vi "界面UI.vi"() -> ()   [LabVIEW 2016, in "科盛超标留样.lvlib"]
uses:
  <vilib>/Utility/miscctls.llb/LVPointTypeDef.ctl
panel:
  in  "当前解析模式":string(combo)
  in  "切换串口":bool
  out "查询系统状态":T1
  out "查询瓶记录":T2
  out "输出数组":T3(array[cluster])
  in  "留样命令":bool
  in  "供样命令":bool
  in  "触发采样":bool
  in  "查询系统状态":bool
  in  "远程取样":bool
  in  "复位指令":bool
  in  "查询瓶记录":bool
  in  "查询采样记录":bool
  in  "VISA resource name":refnum<visa-resource-name>="COM2" caption="VISA资源名称"
  in  "写入缓冲区":string
  out "读取缓冲区":string
  out "source":string
  out "通讯":bool
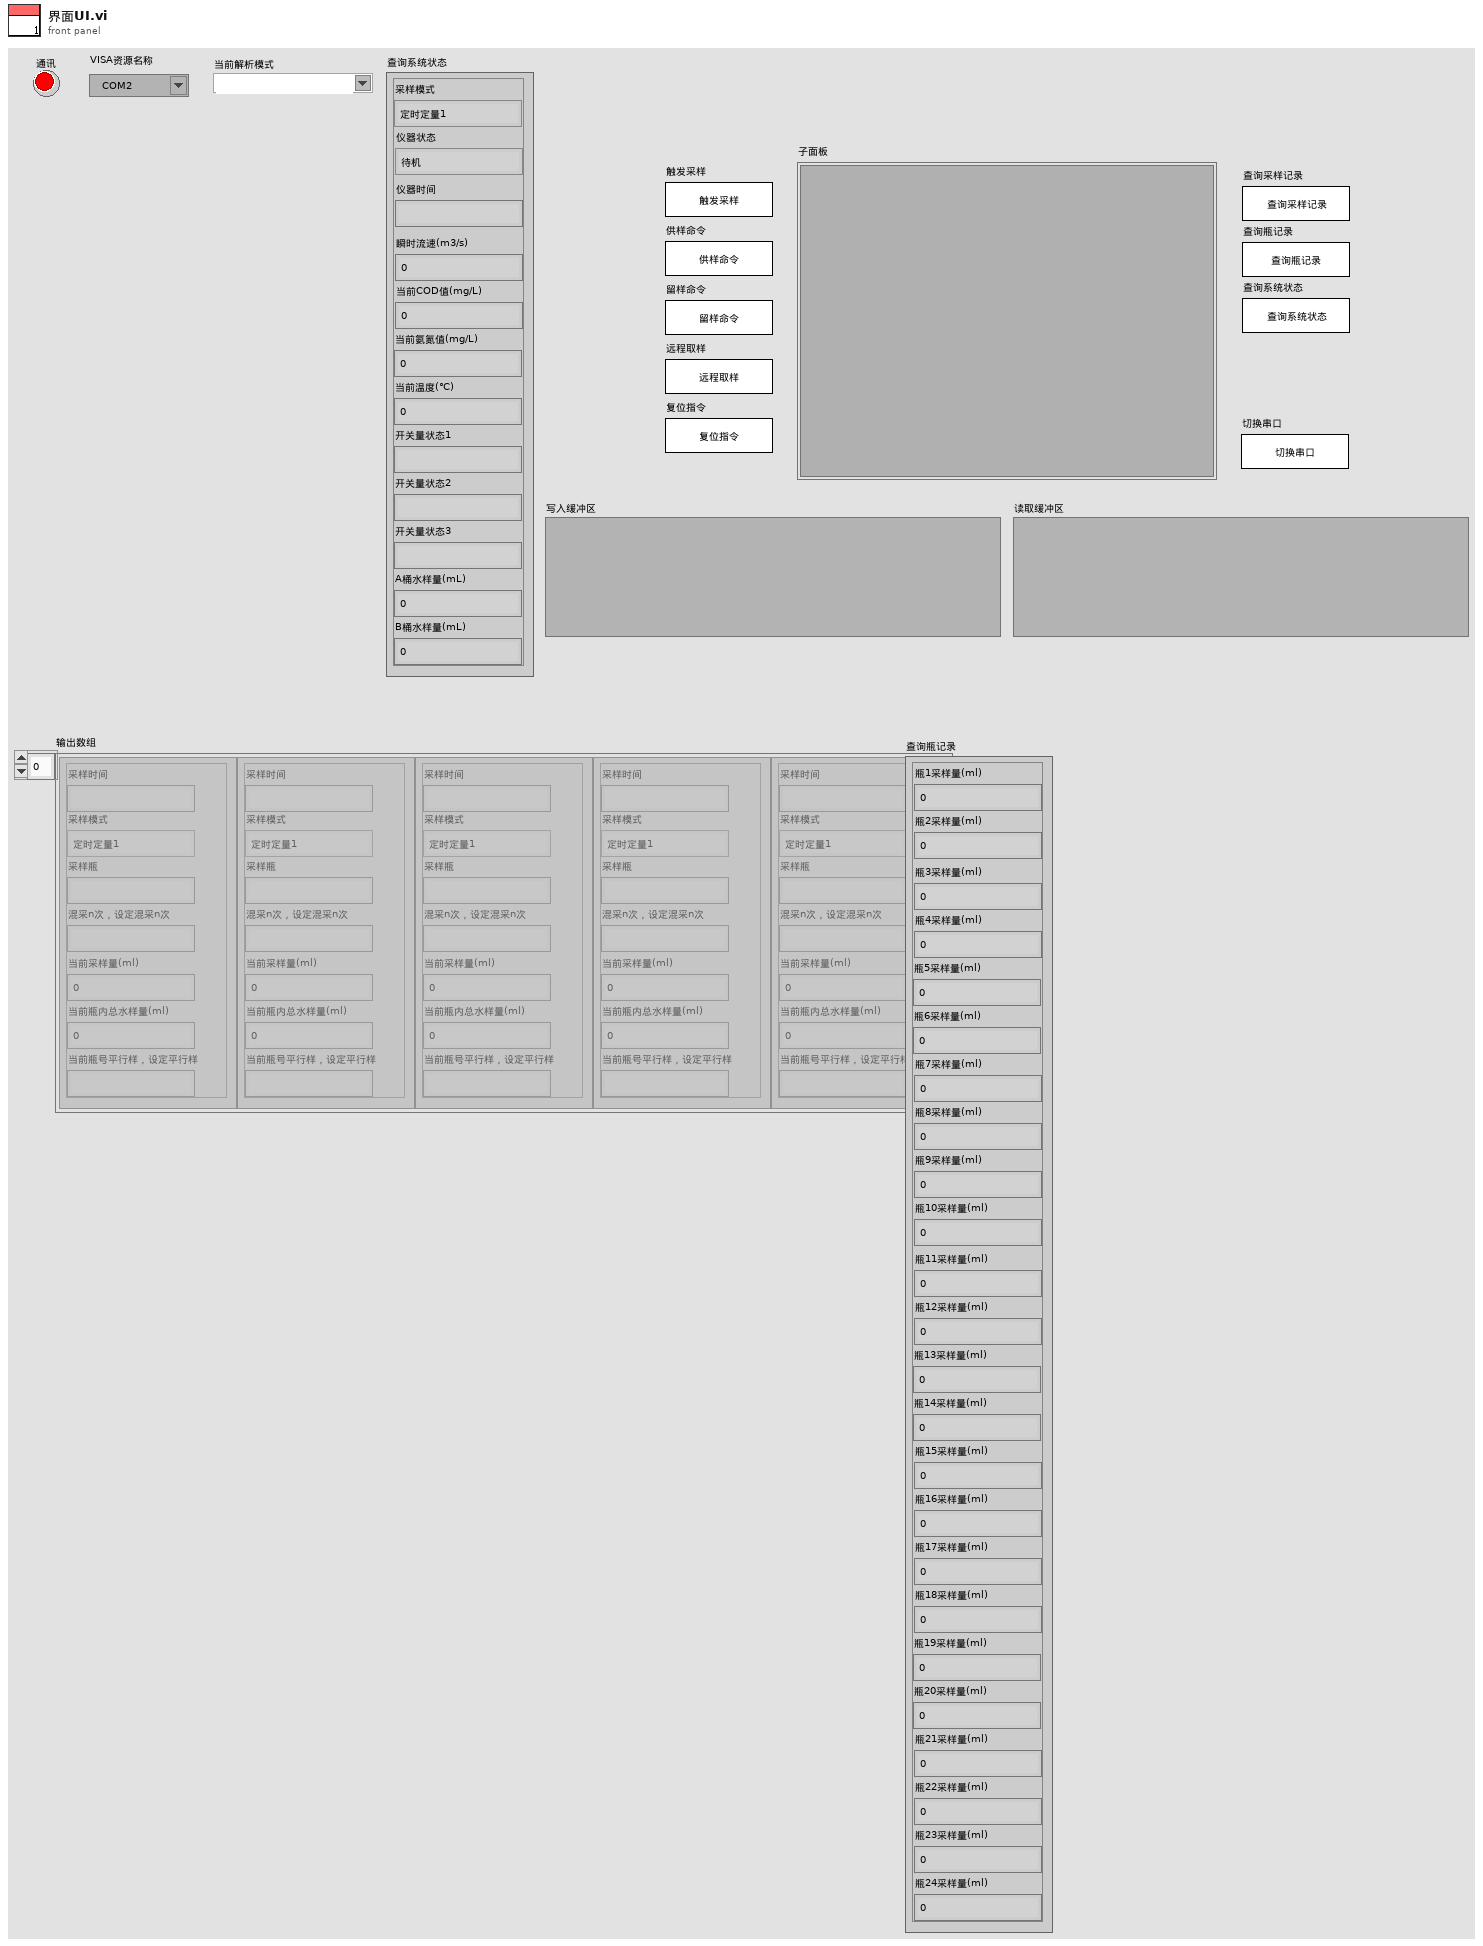
[diagram p1: front panel]
types:
  T1 = cluster{"采样模式":enum16{"定时定量1", "定时定量2", "定流定量", "定时比例", "同步留样", "超标留样", "触发采样", "定时采样1", "定流供样", "定时采样2", "远程取样", "手动取样", "流量跟踪"}, "仪器状态":enum16{"待机", "运行中"}, "仪器时间":string, "瞬时流速(m3/s)":dbl, "当前COD值(mg/L)":dbl, "当前氨氮值(mg/L)":dbl, "当前温度(℃)":dbl, "开关量状态1":string, "开关量状态2":string, "开关量状态3":string, "A桶水样量(mL)":dbl, "B桶水样量(mL)":dbl}
  T2 = cluster{"瓶1采样量(ml)":dbl, "瓶2采样量(ml)":dbl, "瓶3采样量(ml)":dbl, "瓶4采样量(ml)":dbl, "瓶5采样量(ml)":dbl, "瓶6采样量(ml)":dbl, "瓶7采样量(ml)":dbl, "瓶8采样量(ml)":dbl, "瓶9采样量(ml)":dbl, "瓶10采样量(ml)":dbl, "瓶11采样量(ml)":dbl, "瓶12采样量(ml)":dbl, "瓶13采样量(ml)":dbl, "瓶14采样量(ml)":dbl, "瓶15采样量(ml)":dbl, "瓶16采样量(ml)":dbl, "瓶17采样量(ml)":dbl, "瓶18采样量(ml)":dbl, "瓶19采样量(ml)":dbl, "瓶20采样量(ml)":dbl, "瓶21采样量(ml)":dbl, "瓶22采样量(ml)":dbl, "瓶23采样量(ml)":dbl, "瓶24采样量(ml)":dbl}
  T3 = cluster{"采样时间":string, "采样模式":enum16{"定时定量1", "定时定量2", "定流定量", "定时比例", "同步留样", "超标留样", "触发采样", "定时采样1", "定流供样", "定时采样2", "远程取样", "手动取样", "流量跟踪"}, "采样瓶":string, "混采n次，设定混采n次":string, "当前采样量(ml)":dbl, "当前瓶内总水样量(ml)":dbl, "当前瓶号平行样，设定平行样":string}[]
  T4 = enum16{"触发采样", "供样命令", "留样命令", "远程取样", "复位指令", "查询采样记录", "查询瓶记录", "查询系统状态"}
  T5 = typedef "LVPointTypeDef.ctl" = cluster{"Horizontal":i16, "Vertical":i16}
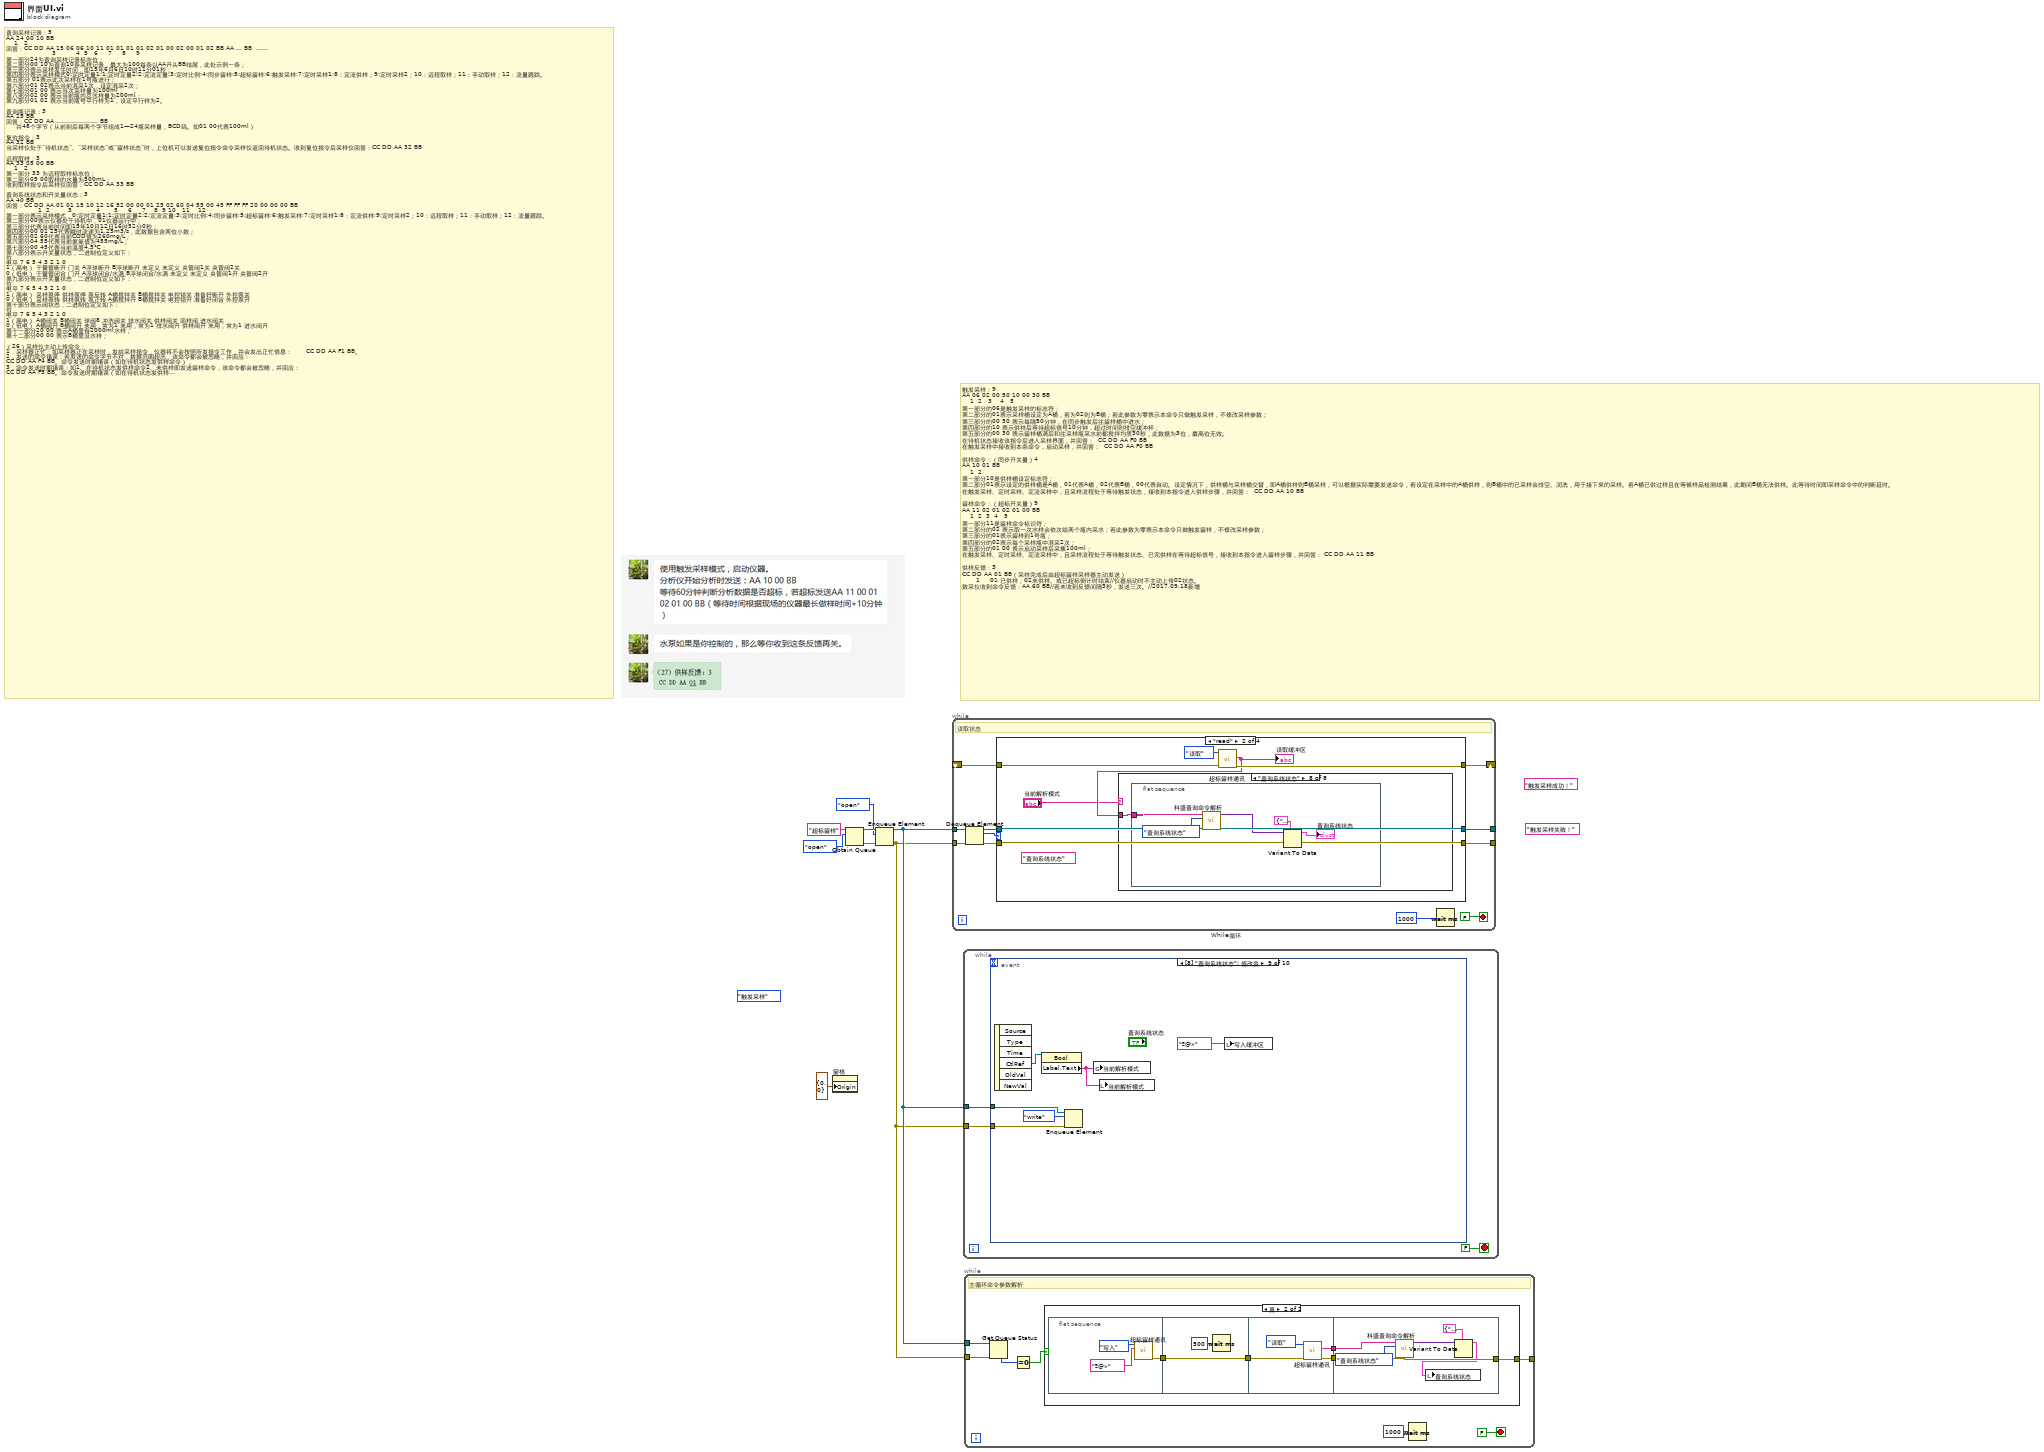
[diagram p0: block diagram]
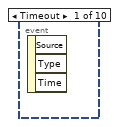
[diagram p3: hidden frame]
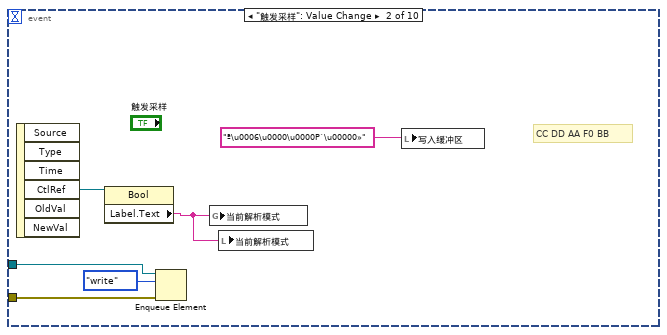
[diagram p4: hidden frame]
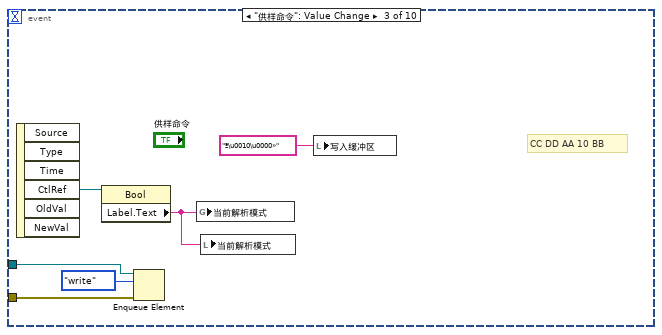
[diagram p5: hidden frame]
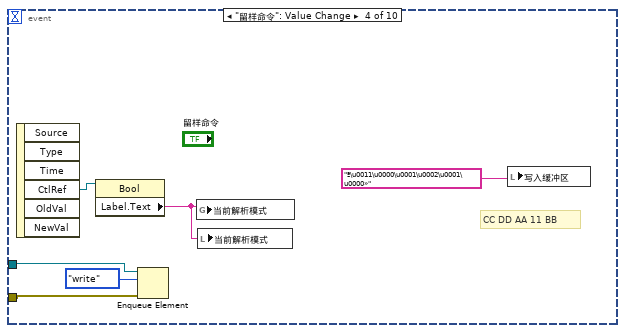
[diagram p6: hidden frame]
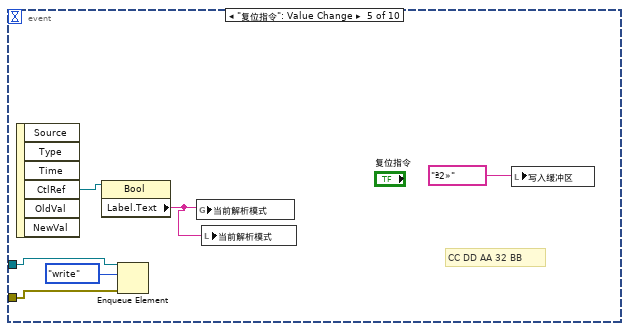
[diagram p7: hidden frame]
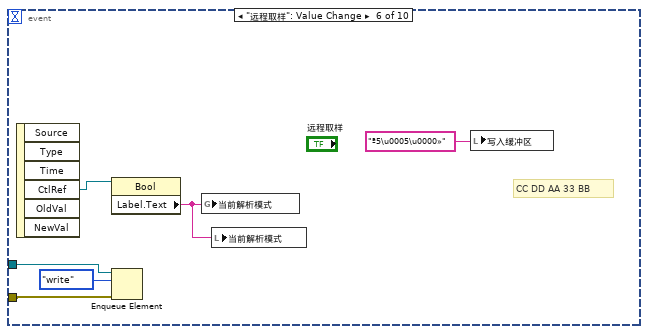
[diagram p8: hidden frame]
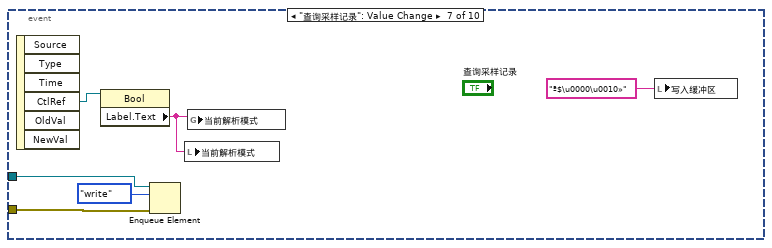
[diagram p9: hidden frame]
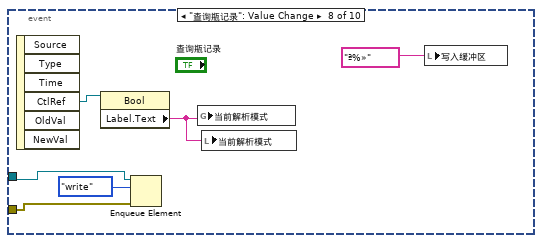
[diagram p10: hidden frame]
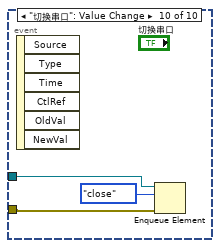
[diagram p11: hidden frame]
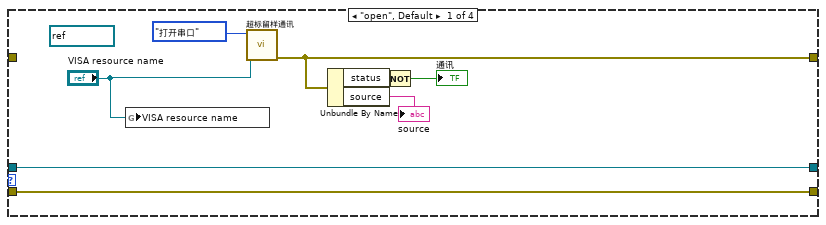
[diagram p12: hidden frame]
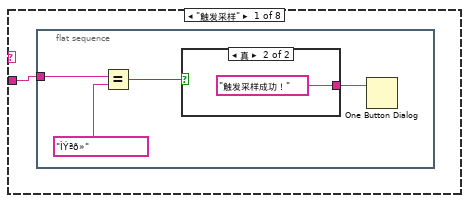
[diagram p13: hidden frame]
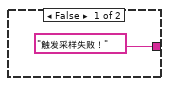
[diagram p14: hidden frame]
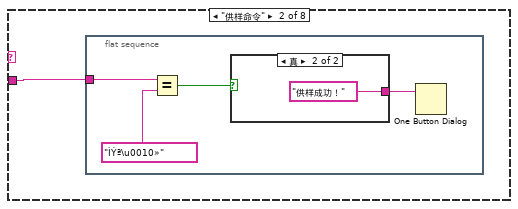
[diagram p15: hidden frame]
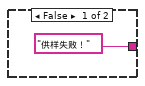
[diagram p16: hidden frame]
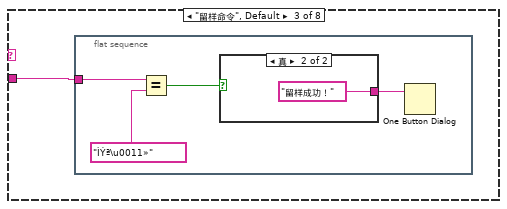
[diagram p17: hidden frame]
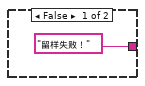
[diagram p18: hidden frame]
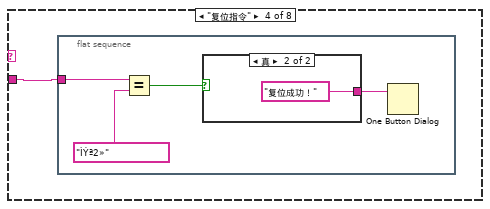
[diagram p19: hidden frame]
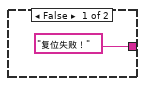
[diagram p20: hidden frame]
diagram:
  (unwired) "触发采样成功！" ("消息")
  (unwired) "触发采样失败！" ("消息")
  (unwired) T4."触发采样" ("功能输入")
  # "查询采样记录：5\nAA 24 00 10 BB\n    1   2\n回答：CC DD AA 15 06 06 10 11 01 01 01 01 02 01 00 02 00 01 02 BB AA ... BB  ......\n                       3          4  5   6     7     8     9\n第一部分24为查询采样记录标志位；\n第二部分00 10为查询10条采样记录，最大为100每条以AA开头BB结尾，此处示例一条；\n第三部分表示采样发生时间，即15年6月6日10时11分01秒；\n第四部分表示采样模式0:定时定量1;1:定时定量2;2:定流定量;3:定时比例;4:同步留样;5:超标留样;6:触发采样;7:定时采样1;8：定流供样；9:定时采样2；10：远程取样；11：手动取样；12：流量跟踪。\n第五部分 01表示此次采样在1号瓶进行；\n第六部分01 02表示当前混采1次，设定混采2次；\n第七部分01 00 表示当次采样量为100ml；\n第八部分02 00 表示当前瓶内总水样量为200ml；\n第九部分01 02 表示当前瓶号平行样为1，设定平行样为2。\n\n查询瓶记录：3\nAA 25 BB\n回答：CC DD AA ………………… BB\n     共48个字节（从前到后每两个字节组成1—24瓶采样量，BCD码。如01 00代表100ml）\n\n复位指令：3\nAA 32 BB\n当采样仪处于“待机状态”、“采样状态”或“留样状态”时，上位机可以发送复位指令命令采样仪返回待机状态。收到复位指令后采样仪回答：CC DD AA 32 BB\n\n远程取样：3\nAA 33 05 00 BB\n    1   2\n第一部分 33 为远程取样标志位；\n第二部分05 00取样的水量为500mL；\n收到取样指令后采样仪回答：CC DD AA 33 BB\n\n查询系统状态和开关量状态：3\nAA 40 BB\n回答：CC DD AA 01 01 15 10 12 16 52 00 00 01 25 02 60 04 55 00 45 FF FF FF 20 00 00 00 BB \n                1  2         3            4       5     6     7    8  9 10   11    12  \n第一部分表示采样模式，0:定时定量1;1:定时定量2;2:定流定量;3:定时比例;4:同步留样;5:超标留样;6:触发采样;7:定时采样1;8：定流供样;9:定时采样2；10：远程取样；11：手动取样；12：流量跟踪。\n第二部分00表示仪器处于待机中，01仪器运行中；\n第三部分代表当前时间即15年10月12日16时52分0秒； \n第四部分00 01 25代表瞬时流速为1.25m3/s，此数据包含两位小数；\n第五部分02 60代表当前COD值为260mg/L；\n第六部分04 55代表当前氨氮值为455mg/L；\n第七部分00 45代表当前温度4.5℃；\n第八部分表示开关量状态，二进制位定义如下：\n位\n电平\t7\t6\t5\t4\t3\t2\t1\t0\n1（高电）\t干簧管断开\t门关\tA浮球断开\tB浮球断开\t未定义\t未定义\t夹管阀1关\t夹管阀2关\n0（低电）\t干簧管闭合\t门开\tA浮球闭合/水满\tB浮球闭合/水满\t未定义\t未定义\t夹管阀1开\t夹管阀2开\n第九部分表示开关量状态，二进制位定义如下：\n位\n电平\t7\t6\t5\t4\t3\t2\t1\t0\n1（高电）\t采样泵停\t供样泵停\t泵反转\tA桶搅拌关\tB桶搅拌关\t电控锁关\t准备好断开\t外控泵关\n0（低电）\t采样泵转\t供样泵转\t泵正转\tA桶搅拌开\tB桶搅拌关\t电控锁开\t准备好闭合\t外控泵开\n第十部分表示阀状态，二进制位定义如下：\n位\n电平\t7\t6\t5\t4\t3\t2\t1\t0\n1（高电）\tA桶阀关\tB桶阀关\t球阀8\t冲洗阀关\t排水阀关\t供样阀关\t回样阀\t进水阀关\n0（低电）\tA桶阀开\tB桶阀开\t未用，常为1\t未用，常为1\t排水阀开\t供样阀开\t未用，常为1\t进水阀开\n第十一部分20 00 表示A桶里有2000ml水样；\n第十二部分00 00 表示B桶里没水样；\n\n（26）采样仪主动上传命令：\n1．采样器正忙：如采样器正在采样时，发给采样指令，仪器将不会按照所发指令工作，并会发出正忙信息：\t\t     CC DD AA F1 BB。\n2．发送的命令错误：若发送的命令字节不对，数据范围超出，该命令都会被忽略，并回应：\nCC DD AA F4 BB。命令发送时期错误（如在待机状态发供样命令），\n3．命令发送时期错误：如1、在待机状态发供样命令2、未供样即发送留样命令，该命令都会被忽略，并回应：\nCC DD AA F5 BB。命令发送时期错误（如在待机状态发供样命令），\n \t4．系统切换进入忙状态：仪器主动上传CC DD AA F6 BB。\n5．系统切换进入空闲状态：仪器主动上传CC DD AA F7 BB。"
  # "触发采样：9\nAA 06 02 00 50 10 00 30 BB\n    1  2   3    4   5         \n第一部分的06是触发采样的标志符；\n第二部分的01表示采样桶设定为A桶，若为02则为B桶；若此参数为零表示本命令只做触发采样，不修改采样参数；\n第三部分的00 50 表示每隔50分钟，在同步触发后往留样桶中进水；\n第四部分的10 表示供样后等待超标信号10分钟，超过时间则排空缓冲杯；\n第五部分的00 30 表示留样桶满后和往采样瓶采水前都搅拌均质30秒，此数据为3位，最高位无效。\n在待机状态接收该指令后进入采样界面，并回答：\t\tCC DD AA F0 BB\n在触发采样中接收到本条命令，启动采样，并回答：\t\tCC DD AA F0 BB\n\n供样命令：（同步开关量）4\nAA 10 01 BB\n    1  2  \n第一部分10是供样桶设定标志符；\n第二部分01表示设定的供样桶是A桶，01代表A桶，02代表B桶，00代表自动。设定情况下，供样桶与采样桶交替，即A桶供样则B桶采样，可以根据实际需要发送命令，若设定在采样中的A桶供样，则B桶中的已采样会排空、润洗，用于接下来的采样。若A桶已供过样且在等候样品检测结果，此期间B桶无法供样。此等待时间即采样命令中的判断延时。\n在触发采样、定时采样、定流采样中，且采样流程处于等待触发状态，接收到本指令进入供样步骤，并回答：\t\tCC DD AA 10 BB\n\n留样命令：（超标开关量）9\nAA 11 02 01 02 01 00 BB\n    1  2  3  4   5    \n第一部分11是留样命令标识符；\n第二部分的02 表示取一次水样会依次给两个瓶内采水；若此参数为零表示本命令只做触发留样，不修改采样参数；\n第三部分的01表示留样到1号瓶；\n第四部分的02表示每个采样瓶中混采2次；\n第五部分的01 00 表示启动采样后采集100ml；\n在触发采样、定时采样、定流采样中，且采样流程处于等待触发状态、已完供样在等待超标信号，接收到本指令进入留样步骤，并回答：\tCC DD AA 11 BB\n\n供样反馈：3\nCC DD AA 01 BB（采样完成后由超标留样采样器主动发送）\n  \t\t   1  \t\t\t01 已供样；02未供样、或已超标倒计时结束//仪器启动时不主动上传02状态。\n数采仪收到命令反馈：AA 60 BB//若未收到反馈间隔3秒，发送三次。//2017.09.18新增"
  n1 = property on="窗格" class="Pane"("Origin"=T5 {"Horizontal"=0, "Vertical"=0} ("原点")) -> ()  [unwired: 2 in, 2 out]
  n2 = Obtain Queue(name (unnamed)="超标留样" ("名称（未命名）"), element data type=enum16{"open", "read", "write", "close"}."open") -> (queue out=w6:refnum<queue>, error out=w5:errorcluster)  [unwired: 3 in, 1 out]
  n3 = Enqueue Element(queue=w6, element=enum16{"open", "read", "write", "close"}."open", error in (no error)=w5) -> (queue out=w3:refnum<queue>, error out=w2:errorcluster)  [unwired: 1 in, 1 out]
  n4 = while "While循环" {
    tunnel: w3 -> [w17]
    tunnel: w2 -> [w16]
    tunnel: [w12] -> _
    tunnel: [w11] -> _
    shift-right: [w10] -> _
    shift-left: _ -> [w9]
    stop <- FALSE stop-if-true
    # "读取状态"
    n5 = Dequeue Element(queue=w17, error in (no error)=w16) -> (queue out=w14:refnum<queue>, element=w15:enum16{"open", "read", "write", "close"}, error out=w13:errorcluster)  [unwired: 1 in, 1 out]
    n6 = case shown="\"read\"" w15 {
      tunnel: [w26 w33 w91 w103] -> w10
      tunnel: w14 -> [w24 w31 w96 w102]
      tunnel: w13 -> [w23 w30 w95 w101]
      tunnel: [w24 w31 w94 w99] -> w12
      tunnel: [w23 w30 w93 w98] -> w11
      tunnel: w9 -> [_ w34 w92 w105]
      frame "open", Default {
        (unwired) refnum<visa-resource-name> "COM2" ("VISA resource name")
        n7 = global write "超标留样全局.vi" "VISA resource name"("VISA resource name") -> ()
        n8 = call "超标留样通讯.vi"("VISA resource name"="VISA resource name", "功能输入"=enum16{"打开串口", "写入", "读取", "关闭串口"}."打开串口") -> ("error out"=w26:errorcluster)  [unwired: 7 in, 2 out]
        n9 = Unbundle By Name(w26) -> ("status"=w21:bool, "source"=→"source":string)
        n10 = Not(x=w21) -> (.not. x?=→"通讯":bool)
      }
      frame "read" {
        (unwired) "查询系统状态" ("当前解析模式")
        n11 = call "超标留样通讯.vi"("error in (no error)"=w34, "功能输入"=enum16{"打开串口", "写入", "读取", "关闭串口"}."读取") -> ("error out"=w33:errorcluster, "读取缓冲区"=w29:string)  [unwired: 7 in, 1 out]
        "读取缓冲区" <- w29
        n12 = case shown="\"查询系统状态\"" "当前解析模式" {
          tunnel: w29 -> [w35 w42 w49 w56 w63 w70 w76 w82]
          frame "触发采样" {
            n13 = flat-sequence {
              tunnel: w35 -> [w39]
              frame #0 {
                n14 = Equal?(x=w39, y="ÌÝªð»") -> (x = y?=w37:bool)
                n15 = case shown="真" w37 {
                  tunnel: ["触发采样失败！" ("消息") "触发采样成功！" ("消息")] -> w36
                  frame False {
                  }
                  frame True {
                  }
                }
                n16 = One Button Dialog(message=w36) -> ()  [unwired: 1 in, 1 out]
              }
            }
          }
          frame "供样命令" {
            n17 = flat-sequence {
              tunnel: w42 -> [w46]
              frame #0 {
                n18 = Equal?(x=w46, y="ÌÝª\u0010»") -> (x = y?=w44:bool)
                n19 = case shown="真" w44 {
                  tunnel: ["供样失败！" ("消息") "供样成功！" ("消息")] -> w43
                  frame False {
                  }
                  frame True {
                  }
                }
                n20 = One Button Dialog(message=w43) -> ()  [unwired: 1 in, 1 out]
              }
            }
          }
          frame "留样命令", Default {
            n21 = flat-sequence {
              tunnel: w49 -> [w53]
              frame #0 {
                n22 = Equal?(x=w53, y="ÌÝª\u0011»") -> (x = y?=w51:bool)
                n23 = case shown="真" w51 {
                  tunnel: ["留样失败！" ("消息") "留样成功！" ("消息")] -> w50
                  frame False {
                  }
                  frame True {
                  }
                }
                n24 = One Button Dialog(message=w50) -> ()  [unwired: 1 in, 1 out]
              }
            }
          }
          frame "复位指令" {
            n25 = flat-sequence {
              tunnel: w56 -> [w60]
              frame #0 {
                n26 = Equal?(x=w60, y="ÌÝª2»") -> (x = y?=w58:bool)
                n27 = case shown="真" w58 {
                  tunnel: ["复位失败！" ("消息") "复位成功！" ("消息")] -> w57
                  frame False {
                  }
                  frame True {
                  }
                }
                n28 = One Button Dialog(message=w57) -> ()  [unwired: 1 in, 1 out]
              }
            }
          }
          frame "远程取样" {
            n29 = flat-sequence {
              tunnel: w63 -> [w67]
              frame #0 {
                n30 = Equal?(x=w67, y="ÌÝª3»") -> (x = y?=w65:bool)
                n31 = case shown="假" w65 {
                  tunnel: ["远程取样失败！" ("消息") "远程取样成功！" ("消息")] -> w64
                  frame False {
                  }
                  frame True {
                  }
                }
                n32 = One Button Dialog(message=w64) -> ()  [unwired: 1 in, 1 out]
              }
            }
          }
          frame "查询采样记录" {
            n33 = flat-sequence {
              tunnel: w70 -> [w75]
              frame #0 {
                n34 = call "科盛查询命令解析.vi"("解析参数选择"=enum16{"查询采样记录", "查询瓶记录", "查询系统状态"}."查询采样记录", "命令输入"=w75) -> ("Variant"=w73:variant)  [unwired: 9 in]
                n35 = Variant To Data(type=T3 [] ("输出数组"), Variant=w73) -> (data=→"输出数组":T3)  [unwired: 1 in, 1 out]
              }
            }
          }
          frame "查询瓶记录" {
            n36 = flat-sequence {
              tunnel: w76 -> [w81]
              frame #0 {
                n37 = call "科盛查询命令解析.vi"("解析参数选择"=enum16{"查询采样记录", "查询瓶记录", "查询系统状态"}."查询瓶记录", "命令输入"=w81) -> ("Variant"=w79:variant)  [unwired: 9 in]
                n38 = Variant To Data(type=T2 {"瓶1采样量(ml)"=0.0, "瓶2采样量(ml)"=0.0, "瓶3采样量(ml)"=0.0, "瓶4采样量(ml)"=0.0, "瓶5采样量(ml)"=0.0, "瓶6采样量(ml)"=0.0, "瓶7采样量(ml)"=0.0, "瓶8采样量(ml)"=0.0, "瓶9采样量(ml)"=0.0, "瓶10采样量(ml)"=0.0, "瓶11采样量(ml)"=0.0, "瓶12采样量(ml)"=0.0, "瓶13采样量(ml)"=0.0, "瓶14采样量(ml)"=0.0, "瓶15采样量(ml)"=0.0, "瓶16采样量(ml)"=0.0, "瓶17采样量(ml)"=0.0, "瓶18采样量(ml)"=0.0, "瓶19采样量(ml)"=0.0, "瓶20采样量(ml)"=0.0, "瓶21采样量(ml)"=0.0, "瓶22采样量(ml)"=0.0, "瓶23采样量(ml)"=0.0, "瓶24采样量(ml)"=0.0} ("查询瓶记录"), Variant=w79) -> (data=→"查询瓶记录":T2)  [unwired: 1 in, 1 out]
              }
            }
          }
          frame "查询系统状态" {
            n39 = flat-sequence {
              tunnel: w82 -> [w87]
              frame #0 {
                n40 = call "科盛查询命令解析.vi"("解析参数选择"=enum16{"查询采样记录", "查询瓶记录", "查询系统状态"}."查询系统状态", "命令输入"=w87) -> ("Variant"=w85:variant)  [unwired: 9 in]
                n41 = Variant To Data(type=T1 {"采样模式"=enum."定时定量1", "仪器状态"=enum."待机", "仪器时间"="", "瞬时流速(m3/s)"=0.0, "当前COD值(mg/L)"=0.0, "当前氨氮值(mg/L)"=0.0, "当前温度(℃)"=0.0, "开关量状态1"="", "开关量状态2"="", "开关量状态3"="", "A桶水样量(mL)"=0.0, "B桶水样量(mL)"=0.0} ("查询系统状态"), Variant=w85) -> (data=→"查询系统状态":T1)  [unwired: 1 in, 1 out]
              }
            }
          }
        }
      }
      frame "write" {
        n42 = call "超标留样通讯.vi"("error in (no error)"=w92, "写入缓冲区"="写入缓冲区", "功能输入"=enum16{"打开串口", "写入", "读取", "关闭串口"}."写入") -> ("error out"=w91:errorcluster)  [unwired: 6 in, 2 out]
        n43 = Enqueue Element(queue=w96, element=enum16{"open", "read", "write", "close"}."read" ("元素"), error in (no error)=w95) -> (queue out=w94:refnum<queue>, error out=w93:errorcluster)  [unwired: 1 in, 1 out]
        n44 = Wait (ms)(milliseconds to wait=u32 500 ("等待时间（毫秒）")) -> ()  [unwired: 1 out]
      }
      frame "close" {
        n45 = call "超标留样通讯.vi"("error in (no error)"=w105, "功能输入"=enum16{"打开串口", "写入", "读取", "关闭串口"}."关闭串口") -> ("error out"=w103:errorcluster)  [unwired: 7 in, 2 out]
        n46 = Enqueue Element(queue=w102, element=enum16{"open", "read", "write", "close"}."open" ("元素"), error in (no error)=w101) -> (queue out=w99:refnum<queue>, error out=w98:errorcluster)  [unwired: 1 in, 1 out]
      }
    }
    n47 = Wait (ms)(milliseconds to wait=u32 1000 ("等待时间（毫秒）")) -> ()  [unwired: 1 out]
  }
  n48 = while {
    tunnel: w3 -> [w107]
    tunnel: w2 -> [w106]
    stop <- FALSE stop-if-true
    n49 = event shown="[8] \"查询系统状态\": 值改变" {
      selector: _ -> [_ _ _ _ _ _ _ _ _ _]
      dyn-events: _ -> [_ _ _ _ _ _ _ _ _ _]
      timeout: _ -> [_ _ _ _ _ _ _ _ _ _]
      tunnel: w107 -> [_ w113 w118 w125 w131 w137 w143 w149 w155 w157]
      tunnel: w106 -> [_ w112 w119 w124 w130 w136 w142 w148 w154 w158]
      event Timeout {
        n50 = event-data() -> ()  [unwired: 1 in, 3 out]
      }
      event "触发采样": Value Change {
        # "CC DD AA F0 BB"
        n51 = event-data() -> ("CtlRef"=w111:refnum<vi>)  [unwired: 1 in, 5 out]
        n52 = property class="Bool"(reference=w111) -> ("Label.Text"=w109:string)  [unwired: 1 in, 2 out]
        n53 = Enqueue Element(queue=w113, element=enum16{"open", "read", "write", "close"}."write" ("元素"), error in (no error)=w112) -> ()  [unwired: 1 in, 3 out]
        n54 = global write "超标留样全局.vi" "当前解析模式"(w109) -> ()
        n55 = local write "当前解析模式"(w109) -> ()
        n56 = local write "写入缓冲区"("ª\u0006\u0000\u0000P`\u00000»" ("写入缓冲区")) -> ()
      }
      event "供样命令": Value Change {
        # "CC DD AA 10 BB"
        n57 = event-data() -> ("CtlRef"=w117:refnum<vi>)  [unwired: 1 in, 5 out]
        n58 = property class="Bool"(reference=w117) -> ("Label.Text"=w115:string)  [unwired: 1 in, 2 out]
        n59 = Enqueue Element(queue=w118, element=enum16{"open", "read", "write", "close"}."write" ("元素"), error in (no error)=w119) -> ()  [unwired: 1 in, 3 out]
        n60 = global write "超标留样全局.vi" "当前解析模式"(w115) -> ()
        n61 = local write "当前解析模式"(w115) -> ()
        n62 = local write "写入缓冲区"("ª\u0010\u0000»" ("写入缓冲区")) -> ()
      }
      event "留样命令": Value Change {
        # "CC DD AA 11 BB"
        n63 = event-data() -> ("CtlRef"=w123:refnum<vi>)  [unwired: 1 in, 5 out]
        n64 = property class="Bool"(reference=w123) -> ("Label.Text"=w121:string)  [unwired: 1 in, 2 out]
        n65 = Enqueue Element(queue=w125, element=enum16{"open", "read", "write", "close"}."write" ("元素"), error in (no error)=w124) -> ()  [unwired: 1 in, 3 out]
        n66 = global write "超标留样全局.vi" "当前解析模式"(w121) -> ()
        n67 = local write "当前解析模式"(w121) -> ()
        n68 = local write "写入缓冲区"("ª\u0011\u0000\u0001\u0002\u0001\u0000»" ("写入缓冲区")) -> ()
      }
      event "复位指令": Value Change {
        # "CC DD AA 32 BB"
        n69 = event-data() -> ("CtlRef"=w129:refnum<vi>)  [unwired: 1 in, 5 out]
        n70 = property class="Bool"(reference=w129) -> ("Label.Text"=w127:string)  [unwired: 1 in, 2 out]
        n71 = Enqueue Element(queue=w131, element=enum16{"open", "read", "write", "close"}."write" ("元素"), error in (no error)=w130) -> ()  [unwired: 1 in, 3 out]
        n72 = global write "超标留样全局.vi" "当前解析模式"(w127) -> ()
        n73 = local write "当前解析模式"(w127) -> ()
        n74 = local write "写入缓冲区"("ª2»" ("写入缓冲区")) -> ()
      }
      event "远程取样": Value Change {
        # "CC DD AA 33 BB"
        n75 = event-data() -> ("CtlRef"=w135:refnum<vi>)  [unwired: 1 in, 5 out]
        n76 = property class="Bool"(reference=w135) -> ("Label.Text"=w133:string)  [unwired: 1 in, 2 out]
        n77 = Enqueue Element(queue=w137, element=enum16{"open", "read", "write", "close"}."write" ("元素"), error in (no error)=w136) -> ()  [unwired: 1 in, 3 out]
        n78 = global write "超标留样全局.vi" "当前解析模式"(w133) -> ()
        n79 = local write "当前解析模式"(w133) -> ()
        n80 = local write "写入缓冲区"("ª5\u0005\u0000»" ("写入缓冲区")) -> ()
      }
      event "查询采样记录": Value Change {
        n81 = event-data() -> ("CtlRef"=w141:refnum<vi>)  [unwired: 1 in, 5 out]
        n82 = property class="Bool"(reference=w141) -> ("Label.Text"=w139:string)  [unwired: 1 in, 2 out]
        n83 = Enqueue Element(queue=w143, element=enum16{"open", "read", "write", "close"}."write" ("元素"), error in (no error)=w142) -> ()  [unwired: 1 in, 3 out]
        n84 = local write "当前解析模式"(w139) -> ()
        n85 = global write "超标留样全局.vi" "当前解析模式"(w139) -> ()
        n86 = local write "写入缓冲区"("ª$\u0000\u0010»" ("写入缓冲区")) -> ()
      }
      event "查询瓶记录": Value Change {
        n87 = event-data() -> ("CtlRef"=w147:refnum<vi>)  [unwired: 1 in, 5 out]
        n88 = property class="Bool"(reference=w147) -> ("Label.Text"=w145:string)  [unwired: 1 in, 2 out]
        n89 = Enqueue Element(queue=w149, element=enum16{"open", "read", "write", "close"}."write" ("元素"), error in (no error)=w148) -> ()  [unwired: 1 in, 3 out]
        n90 = global write "超标留样全局.vi" "当前解析模式"(w145) -> ()
        n91 = local write "当前解析模式"(w145) -> ()
        n92 = local write "写入缓冲区"("ª%»" ("写入缓冲区")) -> ()
      }
      event "查询系统状态": Value Change {
        n93 = event-data() -> ("CtlRef"=w153:refnum<vi>)  [unwired: 1 in, 5 out]
        n94 = property class="Bool"(reference=w153) -> ("Label.Text"=w151:string)  [unwired: 1 in, 2 out]
        n95 = Enqueue Element(queue=w155, element=enum16{"open", "read", "write", "close"}."write" ("元素"), error in (no error)=w154) -> ()  [unwired: 1 in, 3 out]
        n96 = global write "超标留样全局.vi" "当前解析模式"(w151) -> ()
        n97 = local write "当前解析模式"(w151) -> ()
        n98 = local write "写入缓冲区"("ª@»" ("写入缓冲区")) -> ()
      }
      event "切换串口": Value Change {
        n99 = event-data() -> ()  [unwired: 1 in, 6 out]
        n100 = Enqueue Element(queue=w157, element=enum16{"open", "read", "write", "close"}."close" ("元素"), error in (no error)=w158) -> ()  [unwired: 1 in, 3 out]
      }
    }
  }
  n101 = while {
    tunnel: [w164] -> _
    tunnel: w3 -> [w163]
    tunnel: w2 -> [w162]
    stop <- FALSE stop-if-true
    # "主循环命令参数解析"
    n102 = Get Queue Status(queue=w163, error in (no error)=w162) -> (# elements in queue=w161:i32)  [unwired: 1 in, 7 out]
    n103 = Equal To 0?(x=w161) -> (x = 0?=w160:bool)
    n104 = case shown="真" w160 {
      tunnel: [_ w169] -> w164
      frame False {
      }
      frame True {
        n105 = flat-sequence {
          tunnel: [w173] -> w168
          tunnel: w168 -> [w176]
          tunnel: [w176] -> w167
          tunnel: w167 -> [w179]
          tunnel: [w178] -> w171
          tunnel: [w177] -> w170
          tunnel: w171 -> [w186]
          tunnel: w170 -> [w182]
          tunnel: [w186] -> w169
          frame #0 {
            n106 = call "超标留样通讯.vi"("写入缓冲区"="ª@»", "功能输入"=enum16{"打开串口", "写入", "读取", "关闭串口"}."写入") -> ("error out"=w173:errorcluster)  [unwired: 7 in, 2 out]
          }
          frame #1 {
            n107 = Wait (ms)(milliseconds to wait=u32 500 ("等待时间（毫秒）")) -> ()  [unwired: 1 out]
          }
          frame #2 {
            n108 = call "超标留样通讯.vi"("error in (no error)"=w179, "功能输入"=enum16{"打开串口", "写入", "读取", "关闭串口"}."读取") -> ("error out"=w178:errorcluster, "读取缓冲区"=w177:string)  [unwired: 7 in, 1 out]
          }
          frame #3 {
            n109 = call "科盛查询命令解析.vi"("解析参数选择"=enum16{"查询采样记录", "查询瓶记录", "查询系统状态"}."查询系统状态", "命令输入"=w182) -> ("Variant"=w184:variant)  [unwired: 9 in]
            n110 = Variant To Data(type=T1 {"采样模式"=enum."定时定量1", "仪器状态"=enum."待机", "仪器时间"="", "瞬时流速(m3/s)"=0.0, "当前COD值(mg/L)"=0.0, "当前氨氮值(mg/L)"=0.0, "当前温度(℃)"=0.0, "开关量状态1"="", "开关量状态2"="", "开关量状态3"="", "A桶水样量(mL)"=0.0, "B桶水样量(mL)"=0.0} ("查询系统状态"), Variant=w184) -> (data=w181:T1)  [unwired: 1 in, 1 out]
            n111 = local write "查询系统状态"(w181) -> ()
          }
        }
      }
    }
    n112 = Wait (ms)(milliseconds to wait=u32 1000 ("等待时间（毫秒）")) -> ()  [unwired: 1 out]
  }
